vi "Is Default Test.vi"(11 "Int Equal in":refnum<class "Int Equal.lvclass">) -> (2 "Is Default Test?":bool)   [LabVIEW 2018, in "Int Equal.lvclass"]
doc: "For each data type, there should be one class which overrides this vi to define a default test. The default value is false. If no test is set to true, the first test is the default."
uses:
  Int Equal.lvclass
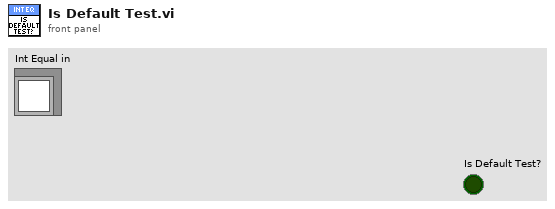
[diagram p1: front panel]
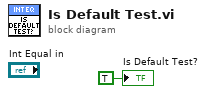
[diagram p0: block diagram]
diagram:
  "Is Default Test?" <- TRUE ("Is Default Test?")
